vi "Lift Control (SubVI).vi"(10 "Buttons":bool[](array[boolean]), 11 "Lift PID gains":T1={"proportional gain (Kc)"=0.8, "integral time (Ti, min)"=0.01, "derivative time (Td, min)"=0.0} {"derivative time (Td, min)" format="%.3f"; "integral time (Ti, min)" format="%.3f"; "proportional gain (Kc)" format="%.3f"}) -> ()   [LabVIEW 2014]
uses:
  <vilib>/Rock Robotics/WPI/Solenoid/WPI_SolenoidValue.ctl
  <vilib>/Rock Robotics/WPI/Solenoid/WPI_SolenoidSetEnum.vi
  <vilib>/addons/control/pid/pid.llb/PID (DBL).vi
  <vilib>/addons/control/pid/NI_PID_pid.lvlib
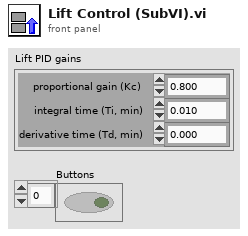
[diagram p1: front panel]
types:
  T1 = cluster{"proportional gain (Kc)":dbl, "integral time (Ti, min)":dbl, "derivative time (Td, min)":dbl}
  T2 = typedef "WPI_SolenoidValue.ctl" = enum16{"Off", "On", "Forward", "Reverse"}
  T3 = typedef "WPI_SwitchDevRef.ctl" = cluster{"DevStatus":errorcluster, "DIO Channel":T4, "Controller":T5, "CntIndex":T6, "Normally Closed":bool}
  T4 = typedef "FPGA_DIOChannel.ctl" = enum8{"DIO 0", "DIO 1", "DIO 2", "DIO 3", "DIO 4", "DIO 5", "DIO 6", "DIO 7", "DIO 8", "DIO 9", "DIO MXP 0", "DIO MXP 1", "DIO MXP 2", "DIO MXP 3", "DIO MXP 4", "DIO MXP 5", "DIO MXP 6", "DIO MXP 7", "DIO MXP 8", "DIO MXP 9", "DIO MXP 10", "DIO MXP 11", "DIO MXP 12", "DIO MXP 13", "DIO MXP 14", "DIO MXP 15", "Invalid"}
  T5 = typedef "FPGA_TypedefDigitalModule.ctl" = enum16{"Controller 1"}
  T6 = typedef "FPGA_CounterCtrSystemIndex.ctl" = enum8{"Ctr 0", "Ctr 1", "Ctr 2", "Ctr 3", "Ctr 4", "Ctr 5", "Ctr 6", "Ctr 7", "Invalid"}
  T7 = typedef "WPI_SolenoidDevRef.ctl" = cluster{"DevStatus":errorcluster, "Pneumatics Control Module":u8, "Forward Solenoid Channel":T8, "Reverse Solenoid Channel":T8}
  T8 = typedef "WPI_SolenoidChannel.ctl" = enum8{"Solenoid 0", "Solenoid 1", "Solenoid 2", "Solenoid 3", "Solenoid 4", "Solenoid 5", "Solenoid 6", "Solenoid 7", "Invalid"}
  T9 = typedef "WPI_MotorControlDeviceRef.ctl" = cluster{"DeviceStatus":errorcluster, "Type":T10, "PWM":cluster{"Controller":T5, "PWM Channel":T11, "DeadBand":T12}, "CAN":cluster{"Device Number":u8, "Control Mode":T13, "Semaphore":T14, "Max Vout":dbl, "TalonSRX Control Mode":T15}, "Invert":bool, "TransformRef":T16, "InvTransformRef":T16}
  T10 = typedef "WPI_MotorControlType.ctl" = enum16{"PWM", "CAN", "CANTalonSRX"}
  T11 = typedef "FPGA_DIOPWMChannel.ctl" = enum8{"PWM 0", "PWM 1", "PWM 2", "PWM 3", "PWM 4", "PWM 5", "PWM 6", "PWM 7", "PWM 8", "PWM 9", "PWM MXP 0", "PWM MXP 1", "PWM MXP 2", "PWM MXP 3", "PWM MXP 4", "PWM MXP 5", "PWM MXP 6", "PWM MXP 7", "PWM MXP 8", "PWM MXP 9", "Invalid"}
  T12 = typedef "WPI_PWMDeadband.ctl" = cluster{"Name":string, "maxPositivePwm":i32, "minPositivePwm":i32, "centerPwm":i32, "maxNegativePwm":i32, "minNegativePwm":i32, "angularRange":u16}
  T13 = typedef "WPI_CANJaguar_ControlMode.ctl" = enum8{"Percent VBus", "Current", "Speed", "Position", "Voltage"}
  T14 = typedef "Semaphore RefNum" = refnum<k1>
  T15 = typedef "WPI_CANTalonSRX_APIControlMode.ctl" = enum8{"Percent VBus", "Speed", "Position", "Slave", "Unchanged / Invalid"}
  T16 = typedef "WPI_PWMTransform_ConPane.ctl" = refnum<vi>
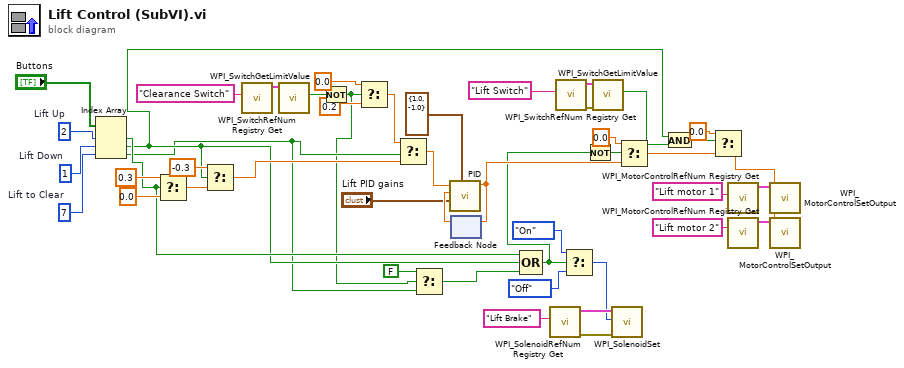
[diagram p0: block diagram]
diagram:
  w47 = 7  # Lift to Clear
  w46 = 1  # Lift Down
  w45 = 2  # Lift Up
  n1 = Index Array(array="Buttons", index #1=w45, index #2=w46, index #3=w47) -> (element #1=w14:bool, element #2=w10:bool, element #3=w6:bool)
  n2 = Select(t=0.3, s=w14, f=0.0) -> (s? t:f=w28:dbl)
  n3 = Select(t=-0.3 ("f"), s=w10, f=w28) -> (s? t:f=w33:dbl)
  n4 = call <vilib>:"WPI_SwitchRefNum Registry Get.vi"("refnum name"="Clearance Switch") -> ("SwitchDevRef"=w8:T3)  [unwired: 9 in, 1 out]
  n5 = call <vilib>:"WPI_SwitchGetLimitValue.vi"("SwitchDevRef"=w8) -> ("Switch Pressed"=w7:bool)  [unwired: 8 in, 2 out]
  n6 = Not(x=w7) -> (.not. x?=w4:bool)
  n7 = Select(t=0.0 ("f"), s=w4, f=0.2 ("t")) -> (s? t:f=w36:dbl)
  n8 = Select(t=w36, s=w6, f=w33) -> (s? t:f=w34:dbl)
  n9 = Select(t=FALSE, s=w4, f=w6) -> (s? t:f=w3:bool)
  n10 = feedback #1() -> (w32:dbl)  [unwired: 1 in]
  n11 = call-poly <vilib>:"PID.vi"("output range"=cluster{"output high":dbl, "output low":dbl} {"output high"=1.0, "output low"=-1.0}, "PID gains"="Lift PID gains", "process variable"=w32, "setpoint"=w34) -> ("output"=w13:dbl)  [unwired: 6 in, 1 out]
  n12 = feedback-in #1(w13) -> ()
  n13 = Compound Arithmetic op=OR(w14, w10, w3) -> (w1:bool)
  n14 = call <vilib>:"WPI_SolenoidRefNum Registry Get.vi"("refnum name"="Lift Brake") -> ("error out"=w19:errorcluster, "SolenoidDevRef"=w18:T7)  [unwired: 9 in]
  n15 = call <vilib>:"WPI_SwitchRefNum Registry Get.vi"("refnum name"="Lift Switch") -> ("error out"=w38:errorcluster, "SwitchDevRef"=w39:T3)  [unwired: 9 in]
  n16 = Select(t=WPI_SolenoidValue."On" ("Value"), s=w1, f=WPI_SolenoidValue."Off" ("Value")) -> (s? t:f=w15:T2)
  n17 = Not(x=w1) -> (.not. x?=w2:bool)
  n18 = call <vilib>:"WPI_SwitchGetLimitValue.vi"("error in (no error)"=w38, "SwitchDevRef"=w39) -> ("Switch Pressed"=w11:bool)  [unwired: 7 in, 2 out]
  n19 = call-poly <vilib>:"WPI_SolenoidSet.vi"("error in (no error)"=w19, "Value"=w15, "SolenoidDevRef"=w18) -> ()  [unwired: 7 in, 2 out]
  n20 = Select(t=0.0, s=w2, f=w13) -> (s? t:f=w41:dbl)
  n21 = And(x=w10, y=w11) -> (x .and. y?=w12:bool)
  n22 = Select(t=0.0, s=w12, f=w41) -> (s? t:f=w42:dbl)
  n23 = call <vilib>:"WPI_MotorControlRefNum Registry Get.vi"("refnum name"="Lift motor 1") -> ("MotorControlDevRef"=w29:T9)  [unwired: 9 in, 1 out]
  n24 = call <vilib>:"WPI_MotorControlRefNum Registry Get.vi"("refnum name"="Lift motor 2") -> ("MotorControlDevRef"=w26:T9)  [unwired: 9 in, 1 out]
  n25 = call <vilib>:"WPI_MotorControlSetOutput.vi"("Output"=w42, "MotorControlDevRef"=w29) -> ()  [unwired: 7 in, 3 out]
  n26 = call <vilib>:"WPI_MotorControlSetOutput.vi"("Output"=w42, "MotorControlDevRef"=w26) -> ()  [unwired: 7 in, 3 out]
